vi "Post-Install Custom Action.vi"(10 "Variant":variant) -> (0 "error out":errorcluster)   [LabVIEW 2014]
uses:
  <vilib>/registry/registry.llb/Registry RtKey.ctl
  <vilib>/AppBuilder/AB_API_Simple/Build (path).vi
  <vilib>/registry/registry.llb/Write Registry Value Simple STR.vi
  <vilib>/AppBuilder/AB_API_Simple/NI_App_Builder_API.lvlib
panel:
  out "concatenated string":string
  out "concatenated string 2":string
  out "dup file":path
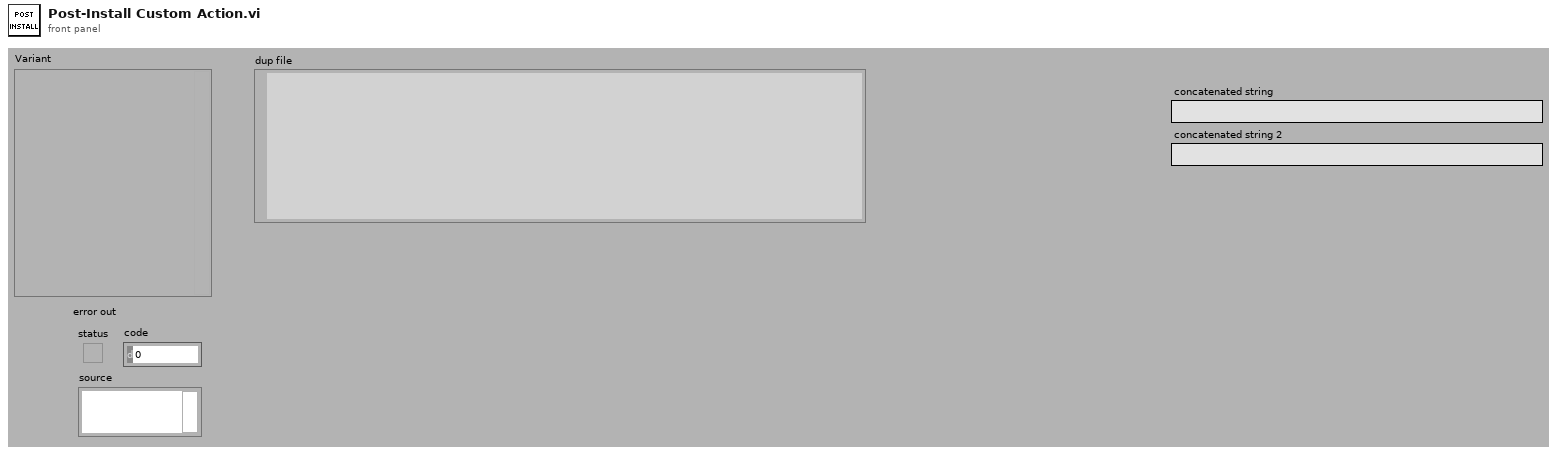
[diagram p1: front panel]
types:
  T1 = typedef "Registry RtKey.ctl" = enum32{"HKEY_CLASSES_ROOT", "HKEY_CURRENT_USER", "HKEY_LOCAL_MACHINE", "HKEY_USERS", "HKEY_PERFORMANCE_DATA", "HKEY_CURRENT_CONFIG", "HKEY_DYN_DATA"}
  T2 = typedef "Registry refnum.ctl" = refnum<k1>
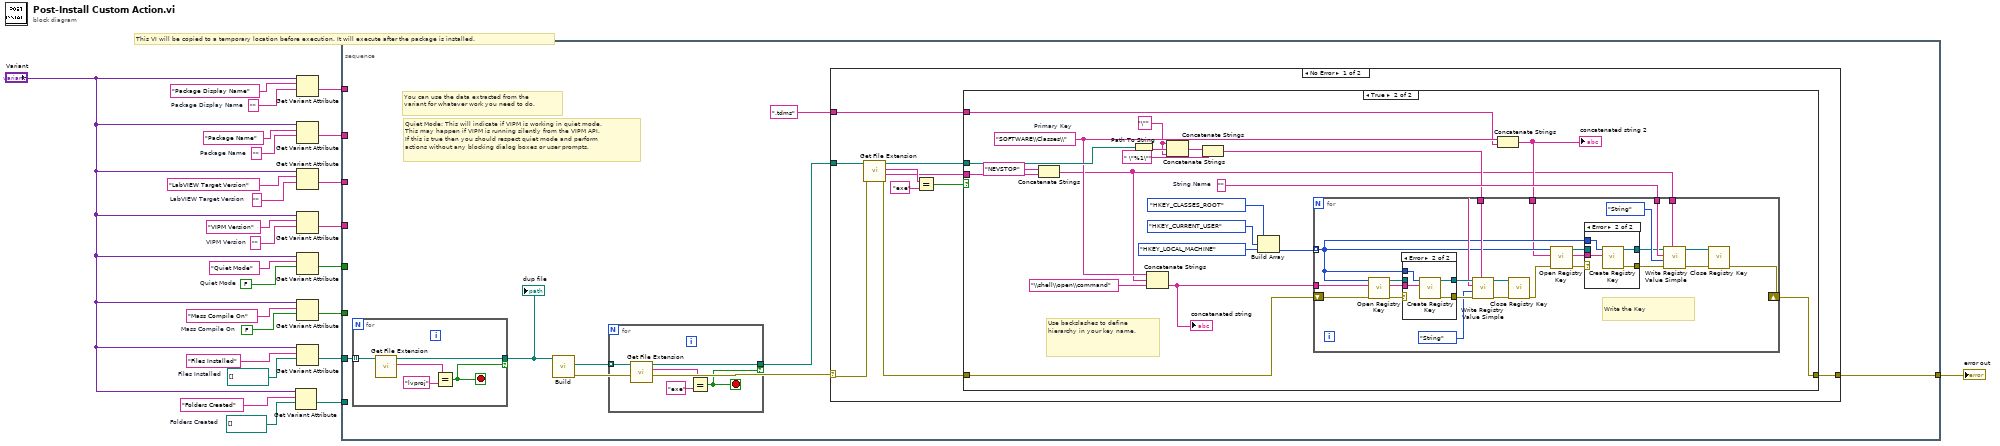
[diagram p0: block diagram]
diagram:
  w2 = path[] []  # Folders Created
  w3 = path[] []  # Files Installed
  w9 = FALSE  # Mass Compile On
  w10 = ""  # Package Display Name
  w17 = FALSE  # Quiet Mode
  w20 = ""  # VIPM Version
  w22 = ""  # LabVIEW Target Version
  w24 = ""  # Package Name
  # "This VI will be copied to a temporary location before execution. It will execute after the package is installed."
  n1 = Get Variant Attribute(Variant="Variant", name="Folders Created", default value (empty Variant)=w2) -> (value=w7:path[])  [unwired: 1 in, 3 out]
  n2 = Get Variant Attribute(Variant="Variant", name="Package Display Name", default value (empty Variant)=w10) -> (value=w16:string)  [unwired: 1 in, 3 out]
  n3 = Get Variant Attribute(Variant="Variant", name="Package Name", default value (empty Variant)=w24) -> (value=w15:string)  [unwired: 1 in, 3 out]
  n4 = Get Variant Attribute(Variant="Variant", name="LabVIEW Target Version", default value (empty Variant)=w22) -> (value=w14:string)  [unwired: 1 in, 3 out]
  n5 = Get Variant Attribute(Variant="Variant", name="VIPM Version", default value (empty Variant)=w20) -> (value=w13:string)  [unwired: 1 in, 3 out]
  n6 = Get Variant Attribute(Variant="Variant", name="Quiet Mode", default value (empty Variant)=w17) -> (value=w12:bool)  [unwired: 1 in, 3 out]
  n7 = Get Variant Attribute(Variant="Variant", name="Mass Compile On", default value (empty Variant)=w9) -> (value=w11:bool)  [unwired: 1 in, 3 out]
  n8 = Get Variant Attribute(Variant="Variant", name="Files Installed", default value (empty Variant)=w3) -> (value=w6:path[])  [unwired: 1 in, 3 out]
  n9 = stacked-sequence {
    tunnel: w16 -> [_]
    tunnel: w15 -> [_]
    tunnel: w14 -> [_]
    tunnel: w13 -> [_]
    tunnel: w12 -> [_]
    tunnel: w11 -> [_]
    tunnel: w6 -> [w32]
    tunnel: w7 -> [_]
    tunnel: [w28] -> w1
    frame #0 {
      # "Quiet Mode: This will indicate if VIPM is working in quiet mode.\nThis may happen if VIPM is running silently from the VIPM API.\nIf this is true then you should respect quiet mode and perform\nactions without any blocking dialog boxes or user prompts."
      # "You can use the data extracted from the variant for whatever work you need to do."
      n10 = for {
        tunnel: w32 -> [w111] mode=indexing
        tunnel: [w110] -> w33 if=w108
        stop <- w108 stop-if-true
        n11 = call <vilib>:"Get File Extension.vi"("file"=w111) -> ("lowercase file extension"=w107:string, "dup file"=w110:path)  [unwired: 7 in, 2 out]
        n12 = Equal?(x=w107, y="lvproj") -> (x = y?=w108:bool)
      }
      "dup file" <- w33
      n13 = call-poly <vilib>:"Build.vi"("Path to project"=w33) -> ("error out"=w29:errorcluster, "Generated files"=w31:path[])  [unwired: 9 in]
      n14 = for {
        tunnel: w31 -> [w106] mode=indexing
        tunnel: [w105] -> w30 if=w103
        stop <- w103 stop-if-true
        n15 = call <vilib>:"Get File Extension.vi"("file"=w106) -> ("lowercase file extension"=w102:string, "dup file"=w105:path)  [unwired: 7 in, 2 out]
        n16 = Equal?(x=w102, y="exe") -> (x = y?=w103:bool)
      }
      n17 = case shown="No Error" w29 {
        selector: w29 -> [w39 w101]
        tunnel: [w43 w101] -> w28
        tunnel: w30 -> [w42 _]
        tunnel: ".tdms" ("string") -> [w34 _]
        frame No Error {
          n18 = call <vilib>:"Get File Extension.vi"("error in (no error)"=w39, "file"=w42) -> ("error out"=w38:errorcluster, "filename without extension"=w35:string, "lowercase file extension"=w36:string, "dup file"=w37:path)  [unwired: 6 in]
          n19 = Equal?(x=w36, y="exe") -> (x = y?=w40:bool)
          n20 = case shown="True" w40 {
            tunnel: [w44 w64] -> w43
            tunnel: w38 -> [w44 w57]
            tunnel: w35 -> [_ w55]
            tunnel: w37 -> [_ w62]
            tunnel: w34 -> [_ w45]
            frame False {
            }
            frame True {
              w49 = "\"" ("string")
              w53 = "SOFTWARE\\Classes\\"  # Primary Key
              w63 = ""  # String Name
              # "Use backslashes to define hierarchy in your key name."
              n21 = Concatenate Strings("NEVSTOP" ("string"), w55) -> (w52:string)
              n22 = Path To String(path=w62) -> (string=w61:string)
              n23 = Concatenate Strings(w53, w52, "\\shell\\open\\command" ("subkey")) -> (w58:string)
              "concatenated string" <- w58
              n24 = Concatenate Strings(w49, w61, w49) -> (w50:string)
              n25 = Concatenate Strings(w50, " \"%1\"" ("string")) -> (w59:string)
              n26 = Build Array(Registry_RtKey."HKEY_CLASSES_ROOT" ("Root Key"), Registry_RtKey."HKEY_CURRENT_USER" ("Root Key"), Registry_RtKey."HKEY_LOCAL_MACHINE" ("Root Key")) -> (w48:T1[])
              n27 = Concatenate Strings(w53, w45) -> (w54:string)
              "concatenated string 2" <- w54
              n28 = for {
                tunnel: w63 -> [w79]
                tunnel: w59 -> [w78]
                tunnel: w58 -> [w77]
                tunnel: w48 -> [w69] mode=indexing
                tunnel: w54 -> [w67]
                tunnel: w52 -> [w66]
                shift-right: [w80] -> w64
                shift-left: w57 -> [w76]
                # "Write the Key"
                n29 = call <vilib>:"Open Registry Key.vi"("error in (no error)"=w76, "subkey"=w77, "root key (HKEY_LOCAL_MACHINE)"=w69) -> ("error out"=w75:errorcluster, "refnum out"=w74:T2)  [unwired: 7 in]
                n30 = case shown="Error" w75 {
                  selector: w75 -> [w96 _]
                  tunnel: [w96 w100] -> w88
                  tunnel: [w95 w99] -> w86
                  tunnel: w69 -> [_ w98]
                  tunnel: w77 -> [_ w97]
                  tunnel: w74 -> [w95 _]
                  frame No Error {
                  }
                  frame Error {
                    n31 = call <vilib>:"Create Registry Key.vi"("subkey"=w97, "root key (HKEY_LOCAL_MACHINE)"=w98) -> ("error out"=w100:errorcluster, "refnum out"=w99:T2)  [unwired: 7 in, 1 out]
                  }
                }
                n32 = call-poly <vilib>:"Write Registry Value Simple.vi"("String/Binary data"=w78, "error in (no error)"=w88, "simple data type"=enum16{"String", "Binary", "DWORD"}."String", "value"=w79, "refnum"=w86) -> ("error out"=w84:errorcluster, "refnum out"=w85:T2)  [unwired: 3 in]
                n33 = call <vilib>:"Close Registry Key.vi"("error in (no error)"=w84, "refnum"=w85) -> ("error out"=w68:errorcluster)  [unwired: 5 in]
                n34 = call <vilib>:"Open Registry Key.vi"("error in (no error)"=w68, "subkey"=w67, "root key (HKEY_LOCAL_MACHINE)"=w69) -> ("error out"=w72:errorcluster, "refnum out"=w73:T2)  [unwired: 7 in]
                n35 = case shown="Error" w72 {
                  selector: w72 -> [w90 _]
                  tunnel: [w90 w94] -> w71
                  tunnel: [w89 w93] -> w70
                  tunnel: w69 -> [_ w92]
                  tunnel: w67 -> [_ w91]
                  tunnel: w73 -> [w89 _]
                  frame No Error {
                  }
                  frame Error {
                    n36 = call <vilib>:"Create Registry Key.vi"("subkey"=w91, "root key (HKEY_LOCAL_MACHINE)"=w92) -> ("error out"=w94:errorcluster, "refnum out"=w93:T2)  [unwired: 7 in, 1 out]
                  }
                }
                n37 = call-poly <vilib>:"Write Registry Value Simple.vi"("String/Binary data"=w66, "error in (no error)"=w71, "simple data type"=enum16{"String", "Binary", "DWORD"}."String", "value"=w79, "refnum"=w70) -> ("error out"=w83:errorcluster, "refnum out"=w82:T2)  [unwired: 3 in]
                n38 = call <vilib>:"Close Registry Key.vi"("error in (no error)"=w83, "refnum"=w82) -> ("error out"=w80:errorcluster)  [unwired: 5 in]
              }
            }
          }
        }
        frame Error {
        }
      }
    }
  }
  "error out" <- w1
